vi "公式复合写入.vi"(8 "公式":cluster{"X^2":dbl, "X":dbl, "b":dbl}, 9 "量程下拉列表":enum16{"低量程", "高量程"}(ring), 10 "测量模式":T1(ring), 11 "参数下拉列表":u16(ring) items=["总氮"=2]) -> ()   [LabVIEW 2016, in "斯坦道总磷.lvlib"]
uses:
  <vilib>/Utility/miscctls.llb/LVPointTypeDef.ctl
panel:
  in  "读取":bool
  in  "一键写入":bool=TRUE
  out "连接的字符串":string
  in  "关闭":bool
  in  "写入":bool
  # "请选择要写入的参数"
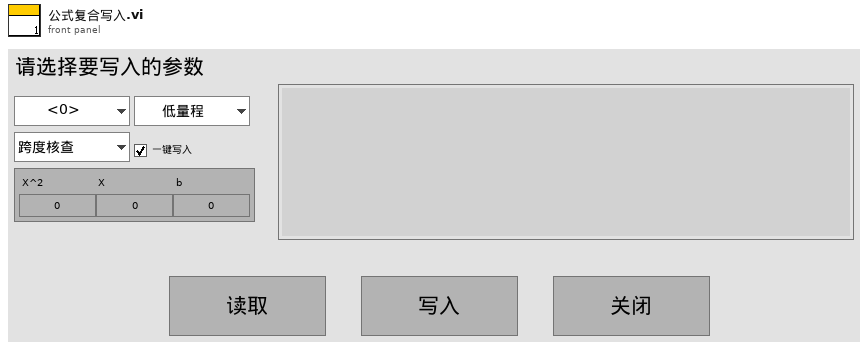
[diagram p1: front panel]
types:
  T1 = enum16{"跨度核查", "水样测量", "零点核查", "标样核查", "加标回收", "快捷测试", "空白校准", "标样校准"}
  T2 = typedef "LVPointTypeDef.ctl" = cluster{"Horizontal":i16, "Vertical":i16}
  T3 = cluster{"系统时间":timestamp, "工作状态":u16, "测量模式":enum16{"待机", "连续模式", "周期模式", "定点模式", "受控模式", "手动模式"}, "告警代码":u16, "故障代码":u16, "日志代码":u16, "软件版本":u16, "F0":sgl, "F1":sgl, "F2":sgl, "F3":sgl, "T":sgl, "H":sgl, "id":u16, "flowid":u16, "量程":u16, "总磷控温温度1":sgl, "营养盐控温温度2":sgl, "ADC":sgl, "结果值":sgl, "运行时间":u16, "步骤详情":string, "步骤流程":string}
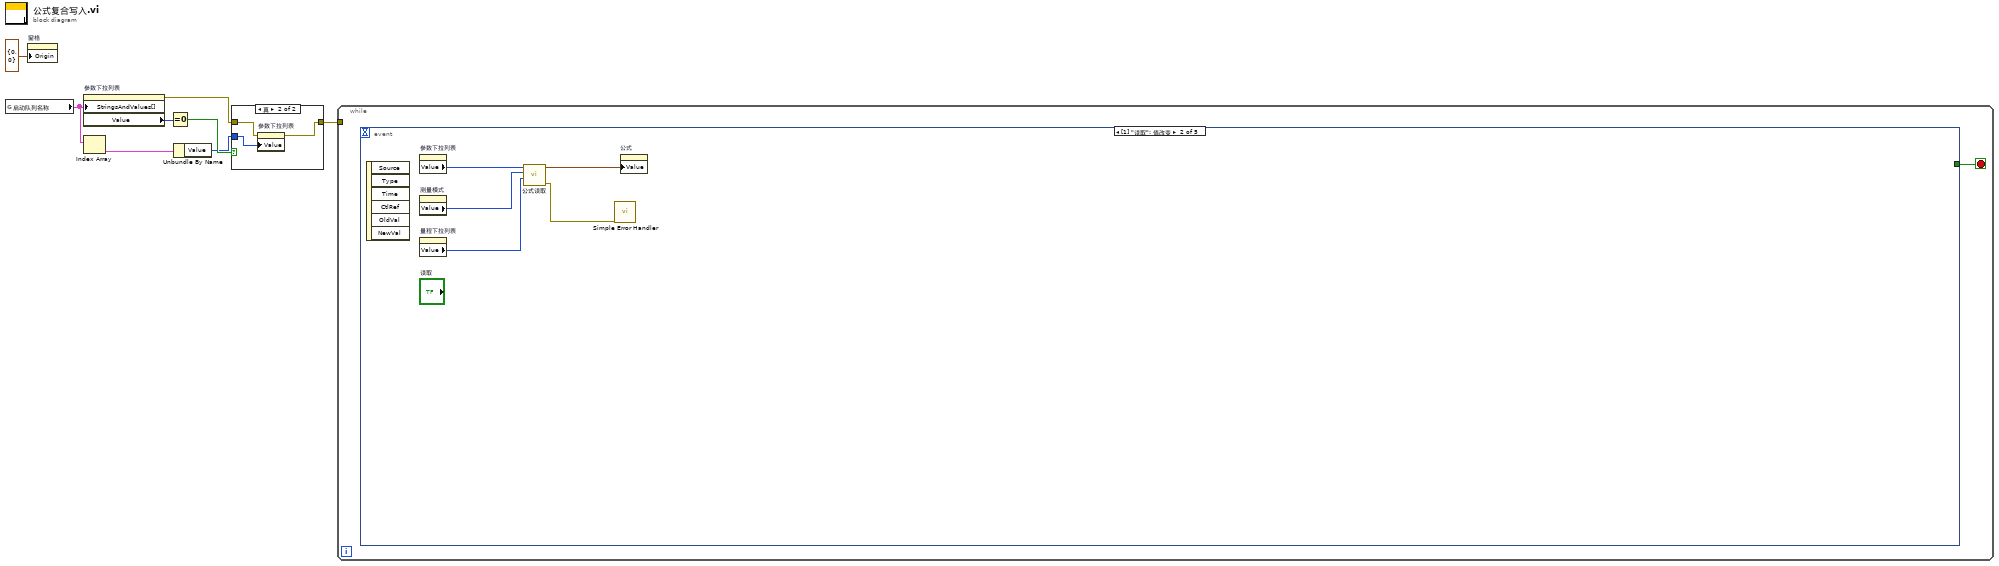
[diagram p0: block diagram]
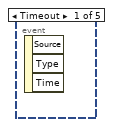
[diagram p3: hidden frame]
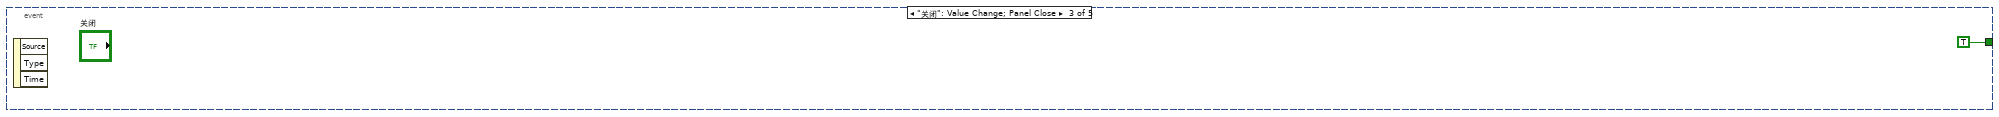
[diagram p4: hidden frame]
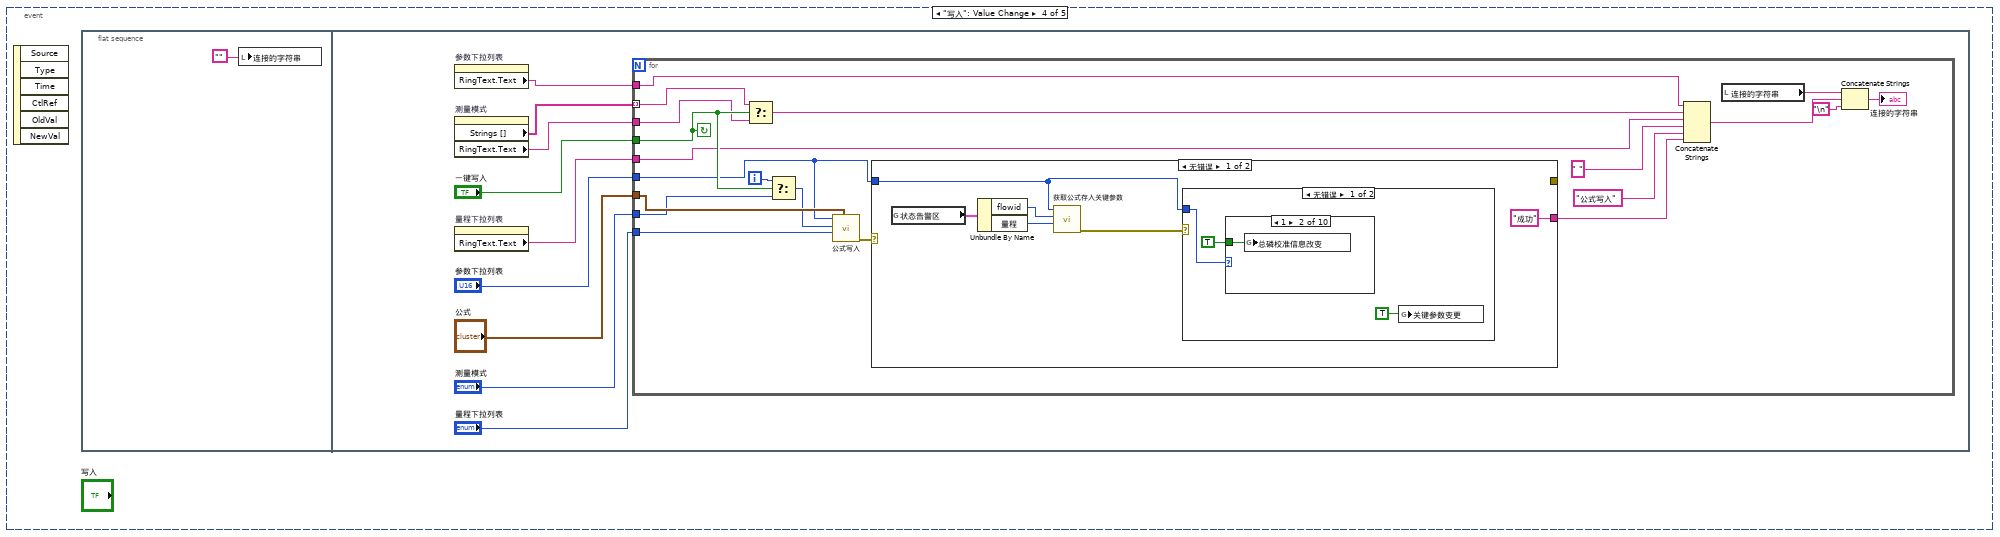
[diagram p5: hidden frame]
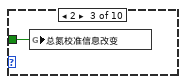
[diagram p7: hidden frame]
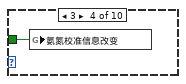
[diagram p8: hidden frame]
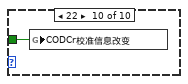
[diagram p14: hidden frame]
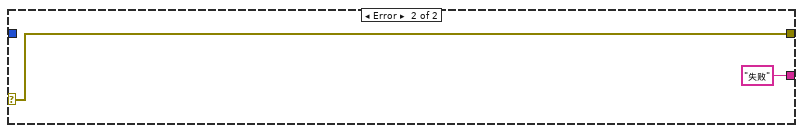
[diagram p16: hidden frame]
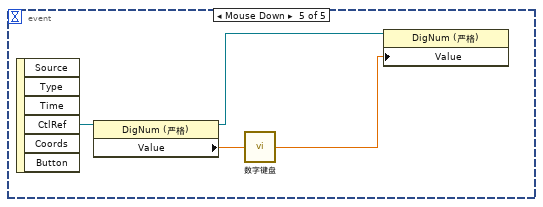
[diagram p17: hidden frame]
diagram:
  n1 = global read "model config var.vi" "启动队列名称"() -> (w3:cluster{"String":string, "Value":u16}[])
  n2 = property on="窗格" class="Pane"("Origin"=T2 {"Horizontal"=0, "Vertical"=0} ("原点")) -> ()  [unwired: 2 in, 2 out]
  n3 = property on="参数下拉列表" class="Ring (严格)"("StringsAndValues[]"=w3) -> (error out=w5:errorcluster, "Value"=w4:u16)  [unwired: 2 in, 1 out]
  n4 = Index Array(array=w3) -> (element=w2:cluster{"String":string, "Value":u16})  [unwired: 1 in]
  n5 = Equal To 0?(x=w4) -> (x = 0?=w7:bool)
  n6 = Unbundle By Name(w2) -> ("Value"=w6:u16)
  n7 = case shown="真" w7 {
    tunnel: w5 -> [w9 w12]
    tunnel: [w9 w11] -> w1
    tunnel: w6 -> [_ w10]
    frame False {
    }
    frame True {
      n8 = property on="参数下拉列表" class="Ring (严格)"(error in=w12, "Value"=w10) -> (error out=w11:errorcluster)  [unwired: 1 in, 1 out]
    }
  }
  n9 = while {
    tunnel: w1 -> [_]
    stop <- w13 stop-if-true
    n10 = event shown="[1] \"读取\": 值改变" {
      selector: _ -> [_ _ _ _ _]
      dyn-events: _ -> [_ _ _ _ _]
      timeout: _ -> [_ _ _ _ _]
      tunnel: [_ _ TRUE _ _] -> w13
      event Timeout {
        n11 = event-data() -> ()  [unwired: 1 in, 3 out]
      }
      event "读取": Value Change {
        n12 = event-data() -> ()  [unwired: 1 in, 6 out]
        n13 = property on="参数下拉列表" class="Ring (严格)"() -> ("Value"=w18:u16)  [unwired: 2 in, 2 out]
        n14 = property on="测量模式" class="Enum (严格)"() -> ("Value"=w17:T1)  [unwired: 2 in, 2 out]
        n15 = property on="量程下拉列表" class="Enum (严格)"() -> ("Value"=w16:enum16{"低量程", "高量程"})  [unwired: 2 in, 2 out]
        n16 = call "公式读取.vi"("量程"=w16, "测量模式"=w17, "测量参数"=w18) -> ("error out"=w14:errorcluster, "公式"=w15:cluster{"X^2":dbl, "X":dbl, "b":dbl})  [unwired: 7 in]
        n17 = call <vilib>:"Simple Error Handler.vi"("error in (no error)"=w14) -> ()  [unwired: 4 in, 5 out]
        n18 = property on="公式" class="Clust (严格)"("Value"=w15) -> ()  [unwired: 2 in, 2 out]
      }
      event "关闭": Value Change; Panel Close {
        n19 = event-data() -> ()  [unwired: 1 in, 3 out]
      }
      event "写入": Value Change {
        n20 = event-data() -> ()  [unwired: 1 in, 6 out]
        n21 = flat-sequence {
          frame #0 {
            n22 = local write "连接的字符串"("") -> ()
          }
          frame #1 {
            n23 = property on="参数下拉列表" class="Ring (严格)"() -> ("RingText.Text"=w22:string)  [unwired: 2 in, 2 out]
            n24 = property on="测量模式" class="Enum (严格)"() -> ("Strings []"=w26:string[], "RingText.Text"=w25:string)  [unwired: 2 in, 2 out]
            n25 = property on="量程下拉列表" class="Enum (严格)"() -> ("RingText.Text"=w21:string)  [unwired: 2 in, 2 out]
            n26 = for {
              tunnel: "公式" -> [w49]
              tunnel: "参数下拉列表" -> [w30]
              tunnel: "量程下拉列表" -> [w48]
              tunnel: w26 -> [w42] mode=indexing
              tunnel: w25 -> [w41]
              tunnel: "一键写入" -> [w43]
              tunnel: "测量模式" -> [w45]
              tunnel: w22 -> [w33]
              tunnel: w21 -> [w31]
              i -> [w46]
              stop <- w43 continue-if-true
              n27 = Select(t=w42, s=w43, f=w41) -> (s? t:f=w35:string)
              n28 = Select(t=w46, s=w43, f=w45) -> (s? t:f=w44:i32)
              n29 = call "公式写入.vi"("公式"=w49, "量程"=w48, "测量模式"=w44, "测量参数"=w30) -> ("error out"=w47:errorcluster)  [unwired: 7 in]
              n30 = case shown="无错误" w47 {
                selector: w47 -> [_ w64]
                tunnel: [_ w64] -> _
                tunnel: ["成功" "失败"] -> w34
                tunnel: w30 -> [w51 _]
                frame No Error {
                  n31 = global read "VAR总磷总氮全局变量.vi" "状态告警区"() -> (w52:T3)
                  n32 = Unbundle By Name(w52) -> ("flowid"=w54:u16, "量程"=w53:u16)
                  n33 = call "获取公式存入关键参数.vi"("量程"=w53, "flowid"=w54, "id"=w51) -> ("error out"=w50:errorcluster)  [unwired: 7 in, 1 out]
                  n34 = case shown="无错误" w50 {
                    tunnel: w51 -> [w56 _]
                    frame No Error {
                      n35 = case shown="1" w56 {
                        tunnel: TRUE ("总磷关键参数改变") -> [_ w59 w60 w61 _ _ _ _ _ w62]
                        frame 0, Default {
                        }
                        frame 1 {
                          n36 = global write "VAR总磷总氮全局变量.vi" "总磷校准信息改变"(w59) -> ()
                        }
                        frame 2 {
                          n37 = global write "VAR总磷总氮全局变量.vi" "总氮校准信息改变"(w60) -> ()
                        }
                        frame 3 {
                          n38 = global write "VAR总磷总氮全局变量.vi" "氨氮校准信息改变"(w61) -> ()
                        }
                        frame 4 {
                        }
                        frame 5 {
                        }
                        frame 6 {
                        }
                        frame 7 {
                        }
                        frame 8 {
                        }
                        frame 22 {
                          n39 = global write "VAR总磷总氮全局变量.vi" "CODCr校准信息改变"(w62) -> ()
                        }
                      }
                      n40 = global write "VAR总磷总氮全局变量.vi" "关键参数变更"(TRUE ("关键参数变更")) -> ()
                    }
                    frame Error {
                    }
                  }
                }
                frame Error {
                }
              }
              n41 = Concatenate Strings(w33, w35, w31, " " ("字符串"), "公式写入", w34) -> (w39:string)
              n42 = local read "连接的字符串"() -> (w36:string)
              n43 = Concatenate Strings(w36, w39, "\n") -> (→"连接的字符串":string)
            }
          }
        }
      }
      event "公式.X^2", "公式.X", "公式.b": Mouse Down {
        n44 = event-data() -> ("CtlRef"=w68:refnum<vi>)  [unwired: 1 in, 5 out]
        n45 = property class="DigNum (严格)"(reference=w68) -> (reference out=w65:refnum<vi>, "Value"=w67:dbl)  [unwired: 1 in, 1 out]
        n46 = call "数字键盘.vi"("OldNumber"=w67) -> ("NewNumber"=w66:dbl)
        n47 = property class="DigNum (严格)"(reference=w65, "Value"=w66) -> ()  [unwired: 1 in, 2 out]
      }
    }
  }
